vi "Client Operation Number.vi"(11 "Client Operation":T1) -> (3 "Op":i32)   [LabVIEW 2020, in "obs-websocket.lvlib"]
uses:
  obs-websocket.lvlib
  Client Operation.ctl
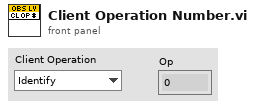
[diagram p1: front panel]
types:
  T1 = typedef "obs-websocket.lvlib/Client Operation.ctl" = enum16{"Identify", "Reidentify", "Request", "RequestBatch"}
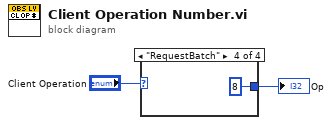
[diagram p0: block diagram]
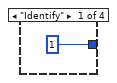
[diagram p2: hidden frame]
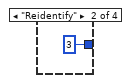
[diagram p3: hidden frame]
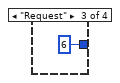
[diagram p4: hidden frame]
diagram:
  n1 = case shown="\"RequestBatch\"" "Client Operation" {
    tunnel: [1 3 6 8] -> w1
    frame "Identify" {
    }
    frame "Reidentify" {
    }
    frame "Request" {
    }
    frame "RequestBatch" {
    }
  }
  "Op" <- w1
